vi "Receive notifier - LiceCam.vi"(10 "Variant":variant, 11 "notifier in":refnum<notifier>) -> (3 "notifier out":refnum<notifier>)   [LabVIEW 2020]
uses:
  <vilib>/userdefined/High Color/IMAQdx.ctl
panel:
  out "Session Out":T1
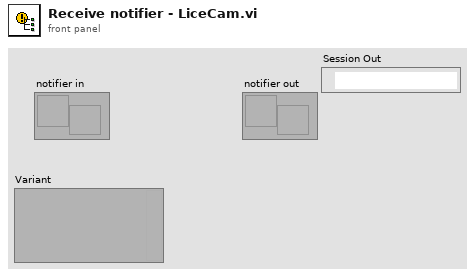
[diagram p1: front panel]
types:
  T1 = typedef "IMAQdx.ctl" = refnum<k21>
  T2 = cluster{"Exposure Time (ms)":u32, "Session Out":T1}
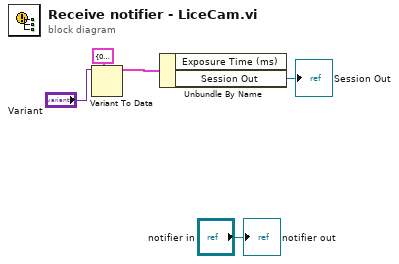
[diagram p0: block diagram]
diagram:
  n1 = Variant To Data(type=T2 {"Exposure Time (ms)"=0, "Session Out"="cam0"} ("Camera Controls"), Variant="Variant") -> (data=w5:T2)  [unwired: 1 in, 1 out]
  n2 = Unbundle By Name(w5) -> ("Session Out"=→"Session Out":T1)  [unwired: 1 out]
  "notifier out" <- "notifier in"
